vi "Get Capacity.vi"(8 "Error In":errorcluster, 11 "ByteBuffer In":refnum<class "ByteBuffer.lvclass">) -> (0 "Error Out":errorcluster, 2 "Capacity":u32, 3 "ByteBuffer Out":refnum<class "ByteBuffer.lvclass">)   [LabVIEW 2015, in "ByteBuffer.lvclass"]
doc: "Returns this buffer's capacity."
uses:
  ByteBuffer.lvclass
  ByteBuffer.lvclass/ByteBuffer.ctl
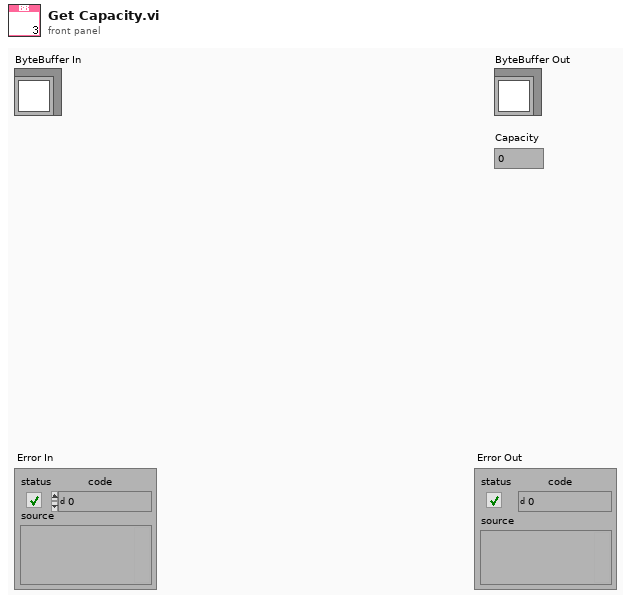
[diagram p1: front panel]
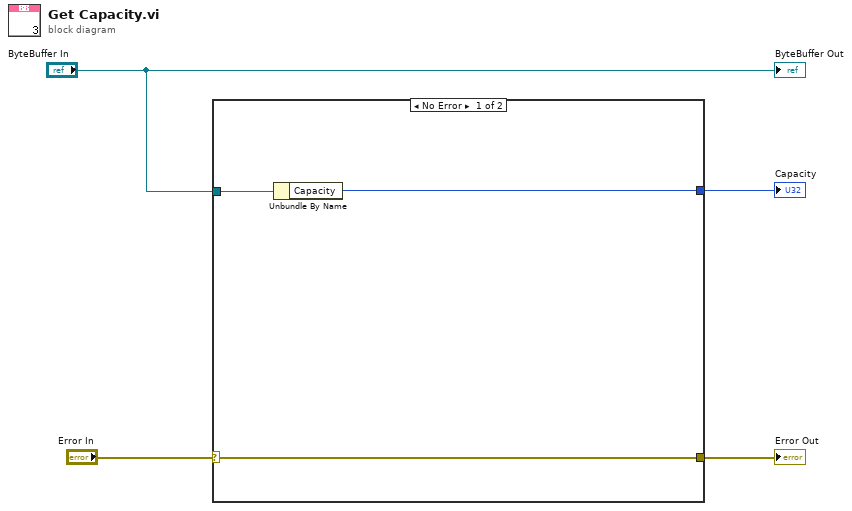
[diagram p0: block diagram]
diagram:
  n1 = case shown="No Error" "Error In" {
    selector: "Error In" -> [w7 w8]
    tunnel: [w7 w8] -> w3
    tunnel: "ByteBuffer In" -> [w6 _]
    tunnel: [w5 _] -> w1
    frame No Error {
      n2 = Unbundle By Name(w6) -> ("Capacity"=w5:u32)
    }
    frame Error {
    }
  }
  "Error Out" <- w3
  "Capacity" <- w1
  "ByteBuffer Out" <- "ByteBuffer In"
